vi "4 Way.vi"() -> ()   [LabVIEW 2012]
uses:
  4 Way Button.ctl
panel:
  in  "Mode Select":enum8{"Off", "Stby", "Hold", "Run"}(ring)
  out "Mode 3":T1
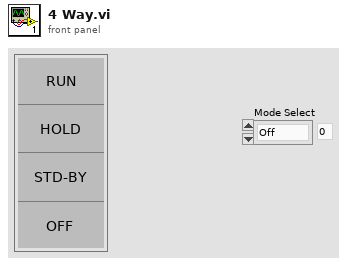
[diagram p1: front panel]
types:
  T1 = typedef "4 Way Button.ctl" = cluster{"Off":bool, "Standby":bool, "Hold":bool, "Run":bool}
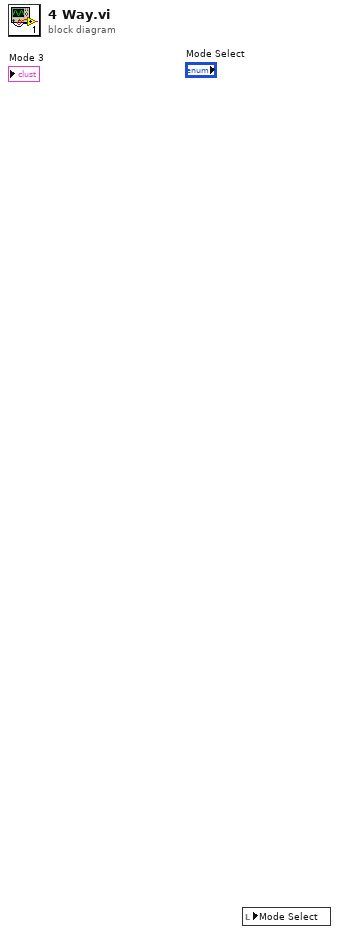
[diagram p0: block diagram]
diagram:
  n1 = local read "Mode Select"() -> ()  [unwired: 1 in]
